vi "normalize pixel.vi"(11 "Input":dbl) -> (3 "Output":dbl)   [LabVIEW 2013]
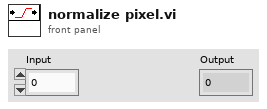
[diagram p1: front panel]
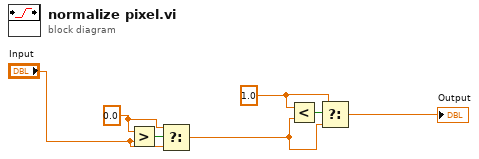
[diagram p0: block diagram]
diagram:
  w5 = 1.0 ("x")
  w2 = 0.0 ("x")
  n1 = Greater?(x=w2, y="Input") -> (0:w7:bool)
  n2 = Select(t=w2, s=w7, f="Input") -> (s? t:f=w4:dbl)
  n3 = Less?(x=w5, y=w4) -> (x < y?=w6:bool)
  n4 = Select(t=w5, s=w6, f=w4) -> (s? t:f=→"Output":dbl)
